vi "BlockAngle.vi"(8 "error in (no error)":errorcluster, 9 "Game ref":refnum<class "Game.lvclass">, 10 "Robot in":refnum<class "Robot.lvclass">, 11 "DefendGoalTactic in":refnum<class "DefendGoalTactic.lvclass">) -> (0 "error out":errorcluster, 2 "Robot out":refnum<class "Robot.lvclass">, 3 "DefendGoalTactic out":refnum<class "DefendGoalTactic.lvclass">)   [LabVIEW 2024, in "DefendGoalTactic.lvclass"]
uses:
  DefendGoalTactic.lvclass
  Game_class/Game.lvclass
  Robot_class/Robot.lvclass
  Game_class/Game.lvclass/Game.ctl
  Object_class/Object.lvclass/Object.ctl
  Team_class/Team.lvclass/Team.ctl
  Field_class/Field.lvclass/Field.ctl
  Robot_class/Robot.lvclass/Robot.ctl
  Game_class/Read BallRef.vi
  Game_class/Read FieldRef.vi
  Game_class/Read DefensiveTeam.vi
  Team_class/Read RobotRef.vi
  Field_class/Read ourGoalPosition.vi
  Object_class/Read position(x,y).vi
  Robot_class/Write dest_orientation.vi
  Robot_class/Write dest_x.vi
  Robot_class/Write dest_y.vi
  Robot_class/Write kick_x.vi
  Robot_class/Write kick_z.vi
  Ally_class/Ally.lvclass
  C:/Users/ROBOIME2/Documents/SSL ROBOIME/SSL_AI/Team_class/Team.lvclass
  Ball_class/Ball.lvclass
  C:/Users/ROBOIME2/Documents/SSL ROBOIME/SSL_AI/Object_class/Object.lvclass
  Field_class/Field.lvclass
  <vilib>/Analysis/NI_AALPro.lvlib
  Utilities_class/Utilities.lvclass
  <vilib>/Analysis/coordinate.llb/2D Cartesian Coordinate Rotation (Scalar).vi
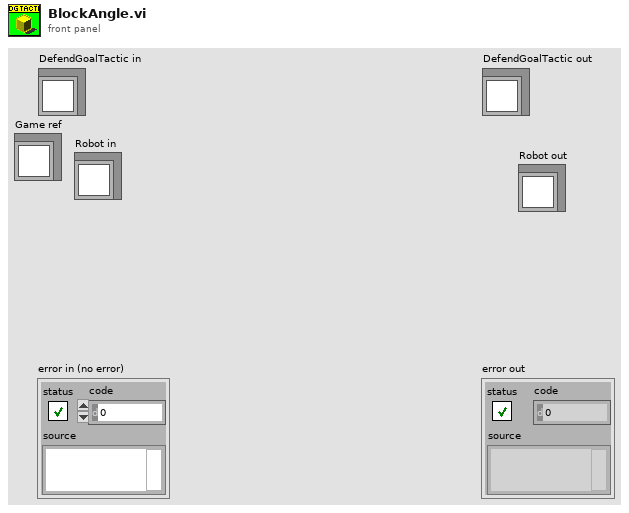
[diagram p1: front panel]
types:
  T1 = typedef "NewParameters.ctl" = cluster{"PenaltyDistance":dbl, "DistanceAttackerToBackBall":dbl, "Division":enum16{"Div B", "Div A"}, "DistanceToAvoidyEnemyRobot":dbl, "BallPlacementDistance":dbl, "DisatanceBehindBallToStealBall":dbl, "MaxDistanceToPositionKickoff":dbl, "BlockEnemyTarget":bool, "MaxStopVAng":dbl, "DistanceMarkerToEnemy":dbl, "IgnoreDribblerContact":bool, "DistanceToBeginEnemyPosession":dbl, "GoToBallWhenEnemyNotMoving":bool, "EnemyDistanceToReduceVelocity":dbl, "TurnOnEnemyDistanceToReduceVelocity":bool, "EnemyDistanceToShootOutBall":dbl, "DefenseKickBall":bool, "MoreKickToGoal? (0-0.3)":dbl, "ChipKickInEnemyField":bool, "ShootOutRobotId":dbl, "FieldLenghtDenominatorInShootOut":dbl, "AdjustPositionInBallPlacement":bool, "PowerGodPass":dbl, "VelocityAbortEnemyPos":dbl, "MaxDistToBeginPass":dbl, "MinDistToBeginPass":dbl, "VelocityInDirects":dbl, "BadDribblerIDs":i32[], "NewKickToDistanceAroundBall":dbl, "PowerAvoidColisionMarker":dbl, "DistanceToAvoidColisionMarker":dbl, "AvoidBallKick":dbl, "DistanceTryKick":dbl, "SuicideKickDIstance":dbl, "AdjustFirstKickDistance":dbl, "AvoidAimLessKick":dbl, "DistanceToAvoidyEnemyShootRobot ":dbl, "NumberOfMarkers":dbl, "PotField":bool, "PIDLateral":bool, "MinDistanceFirstKickX":dbl, "MinDistanceFirstKickY":dbl, "FractionOfDistToTouchGround\nAfterChipKick":dbl, "FractionOfKickxWhen\nComposedWithKickz":dbl, "Style":T2, "MoveInTurnState":bool, "DistFromEnemyToConsider\nMoveInTurnState":dbl, "CascadePID":bool, "TurnAroundParameters":cluster{"Radius":dbl, "Multiplier":dbl, "ChordAngle":dbl}, "SafeDriveVel":dbl, "DistanceToGoToBackBall":dbl, "minDistanceToNotFinish\nEnemyPossession":dbl, "OneTouchShot":cluster{"angleFactor":dbl, "maxAngle":dbl, "Attack":bool, "Defense":bool}, "OpenAngleToGoal":cluster{"minAngle":dbl, "maxAngle":dbl, "minEvaluation":dbl}, "ShotInterception":cluster{"shotSpeed":dbl, "minEnemySpeed":dbl, "maxEnemySpeed":dbl, "minEvaluation":dbl}, "AllyTeamArray":T3[], "maxDefendersNumber":i32, "Zone":cluster{"GuardPositionArray":dbl[][], "ZoneMidField":dbl[], "CenterForwardWidth":dbl}, "MinEvaluationToShoot":dbl, "PassInterception":cluster{"maxPassSpeed":dbl, "minPassSpeed":dbl, "minEnemySpeed":dbl, "chipPassDistance":dbl, "chipPassEvaluation":dbl, "minEvaluation":dbl, "maxEnemySpeed":dbl}, "PassDistance":cluster{"maxDistance":dbl, "minDistance":dbl}, "receiverSpeed":dbl, "maxBallSpeed":dbl, "slackTime":dbl, "Turning radius":dbl, "Turning v_ang":dbl, "AlignError":cluster{"Distance":dbl, "Orientation":dbl, "V_norm(m/s)":dbl, "V_ang (rad/s)":dbl}, "RobotRadius":dbl, "KickerDistance":dbl, "keeper angle  to cover goalpost":dbl, "a_slide":dbl, "a_roll":dbl, "k_switch":dbl}
  T2 = typedef "Style.ctl" = enum16{"Insanity", "Offensive", "Defensive"}
  T3 = typedef "AllyTeam.ctl" = enum16{"Keeper", "Defender", "Attacker"}
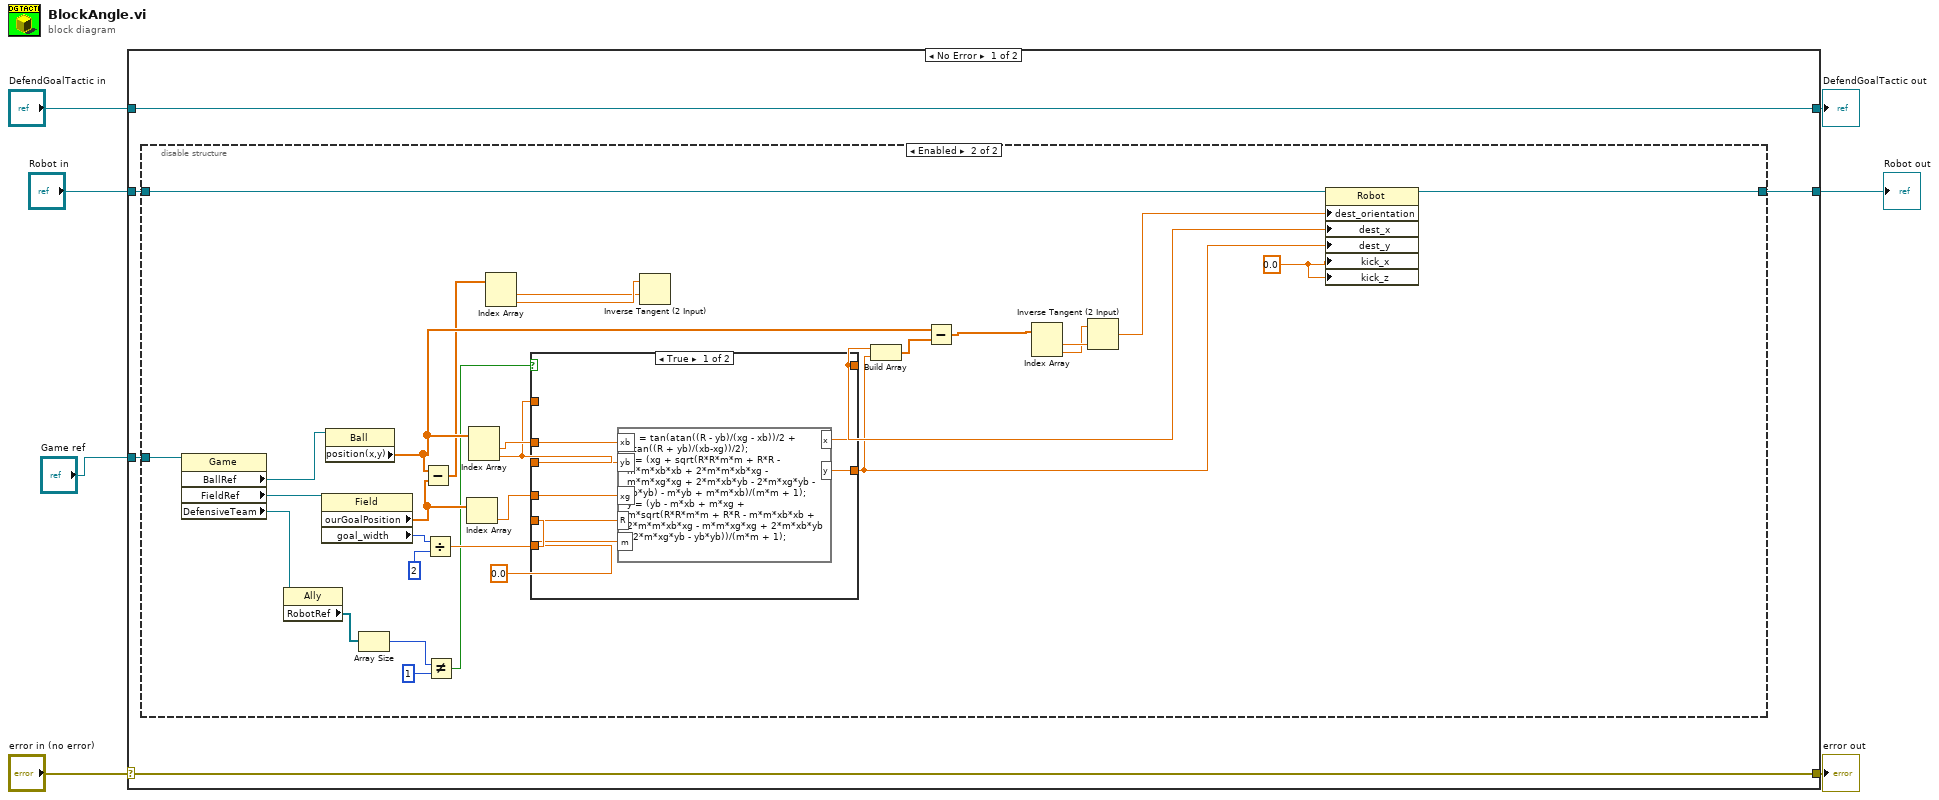
[diagram p0: block diagram]
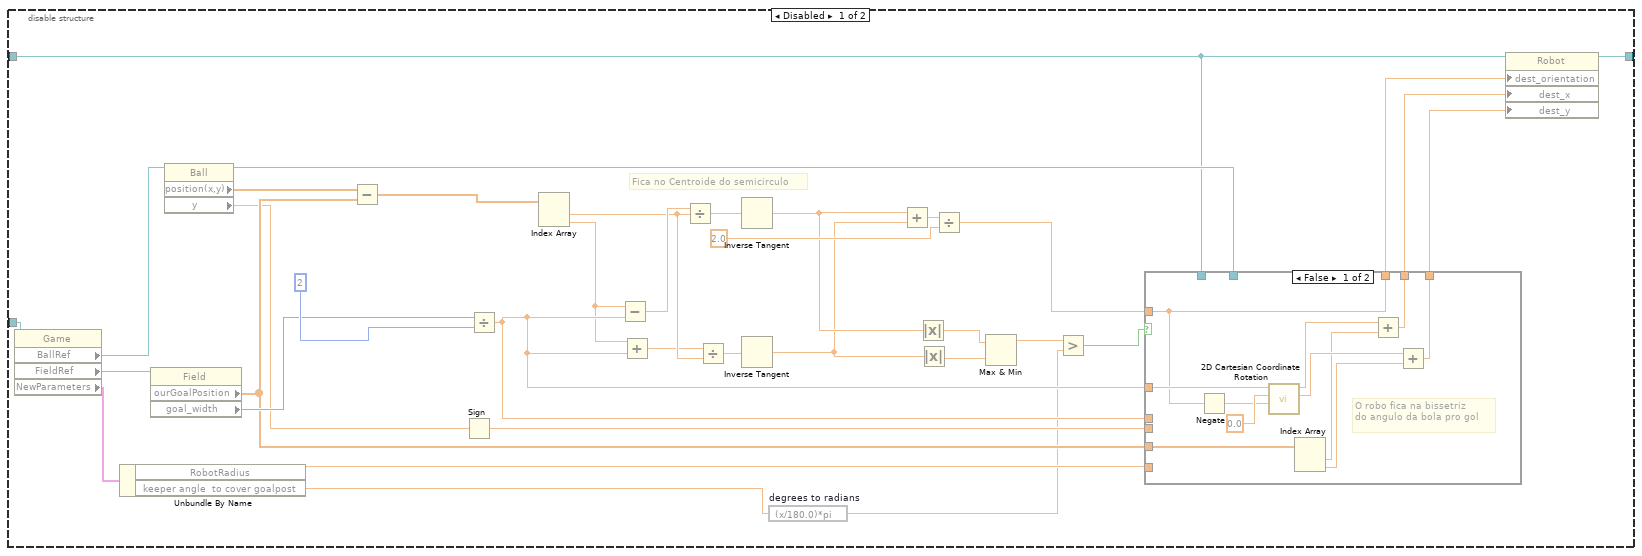
[diagram p2: hidden frame]
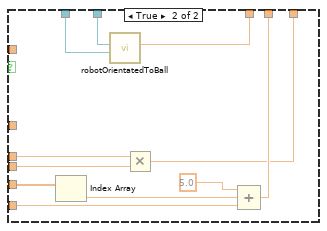
[diagram p3: hidden frame]
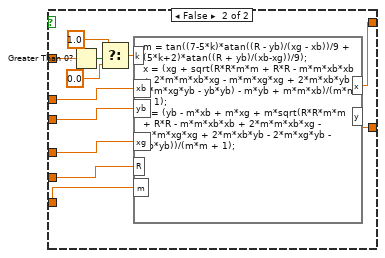
[diagram p4: hidden frame]
diagram:
  n1 = case shown="No Error" "error in (no error)" {
    selector: "error in (no error)" -> [w11 w122]
    tunnel: [w11 w122] -> w6
    tunnel: [w12 w121] -> w4
    tunnel: "DefendGoalTactic in" -> [w12 w121]
    tunnel: "Game ref" -> [w10 _]
    tunnel: "Robot in" -> [w8 w120]
    tunnel: [w9 w120] -> w1
    frame No Error {
      n2 = disable-structure shown="Enabled" {
        disable-tunnel: w10 -> [w23 w100]
        disable-tunnel: [w22 w88] -> w9
        disable-tunnel: w8 -> [w21 w89]
        frame Disabled {
          # "Fica no Centroide do semicirculo"
          n3 = property class="Game"(reference=w23) -> ("BallRef"=w48:refnum<class "Ball.lvclass">, "FieldRef"=w47:refnum<class "Field.lvclass">, "NewParameters"=w29:T1)  [unwired: 1 in, 2 out]
          n4 = Unbundle By Name(w29) -> ("RobotRadius"=w28:dbl, "keeper angle  to cover goalpost"=w13:dbl)
          n5 = property class="Field"(reference=w47) -> ("ourGoalPosition"=w35:dbl[], "goal_width"=w36:i32)  [unwired: 1 in, 2 out]
          n6 = property class="Ball"(reference=w48) -> (reference out=w30:refnum<class "Ball.lvclass">, "position(x,y)"=w46:dbl[], "y"=w25:dbl)  [unwired: 1 in, 1 out]
          n7 = Subtract(x=w46, y=w35) -> (x-y=w44:dbl[])
          n8 = Sign(1:w25) -> (0:w24:dbl)
          n9 = Divide(x=w36, y=2) -> (x/y=w27:dbl)
          n10 = Index Array(array=w44) -> (element #1=w42:dbl, element #2=w26:dbl)  [unwired: 2 in]
          n11 = Subtract(x=w26, y=w27) -> (x-y=w43:dbl)
          n12 = Add(x=w26, y=w27) -> (x+y=w41:dbl)
          n13 = Divide(x=w43, y=w42) -> (x/y=w45:dbl)
          n14 = Divide(x=w41, y=w42) -> (x/y=w40:dbl)
          n15 = Inverse Tangent(1:w45) -> (0:w20:dbl)
          n16 = Inverse Tangent(1:w40) -> (0:w19:dbl)
          n17 = expression code="(x/180.0)*pi" "degrees to radians"(w13) -> (w15:dbl)
          n18 = Add(x=w20, y=w19) -> (x+y=w38:dbl)
          n19 = Absolute Value(x=w20) -> (abs(x)=w18:dbl)
          n20 = Absolute Value(x=w19) -> (abs(x)=w17:dbl)
          n21 = Divide(x=w38, y=2.0) -> (x/y=w32:dbl)
          n22 = Max & Min(x=w18, y=w17) -> (max(x,y)=w16:dbl)  [unwired: 1 out]
          n23 = Greater?(x=w16, y=w15) -> (0:w14:bool)
          n24 = case shown="False" w14 {
            tunnel: w27 -> [w58 _]
            tunnel: w35 -> [w57 w67]
            tunnel: [w51 w64] -> w34
            tunnel: [w50 w61] -> w33
            tunnel: w32 -> [w49 _]
            tunnel: [w49 w69] -> w31
            tunnel: w30 -> [_ w70]
            tunnel: w28 -> [_ w68]
            tunnel: w27 -> [_ w62]
            tunnel: w24 -> [_ w63]
            tunnel: w21 -> [_ w60]
            frame False {
              # "O robo fica na bissetriz \ndo angulo da bola pro gol"
              n25 = Negate(x=w49) -> (-x=w54:dbl)
              n26 = call-poly <vilib>:"2D Cartesian Coordinate Rotation.vi"("theta"=w54, "y"=0.0, "x"=w58) -> ("y out"=w55:dbl, "x out"=w56:dbl)  [unwired: 6 in, 1 out]
              n27 = Index Array(array=w57) -> (element #1=w53:dbl, element #2=w52:dbl)  [unwired: 2 in]
              n28 = Add(x=w56, y=w53) -> (x+y=w51:dbl)
              n29 = Add(x=w55, y=w52) -> (x+y=w50:dbl)
            }
            frame True {
              n30 = Index Array(array=w67) -> (element=w66:dbl)  [unwired: 1 in]
              n31 = call "robotOrientatedToBall.vi"("Robot"=w60, "BallRef"=w70) -> ("Orientation"=w69:dbl)  [unwired: 7 in, 2 out]
              n32 = Multiply(x=w62, y=w63) -> (x*y=w61:dbl)
              n33 = Compound Arithmetic op=ADD(5.0 ("value"), w66, w68) -> (w64:dbl)
            }
          }
          n34 = property class="Robot"(reference=w21, "dest_orientation"=w31, "dest_x"=w34, "dest_y"=w33) -> (reference out=w22:refnum<class "Robot.lvclass">)  [unwired: 1 in, 1 out]
        }
        frame Enabled {
          w83 = 0.0 ("kick_x")
          n35 = property class="Game"(reference=w100) -> ("BallRef"=w98:refnum<class "Ball.lvclass">, "FieldRef"=w99:refnum<class "Field.lvclass">, "DefensiveTeam"=w76:refnum<class "Ally.lvclass">)  [unwired: 1 in, 2 out]
          n36 = property class="Ally"(reference=w76) -> ("RobotRef"=w75:refnum<class "Robot.lvclass">[])  [unwired: 1 in, 2 out]
          n37 = property class="Field"(reference=w99) -> ("ourGoalPosition"=w81:dbl[], "goal_width"=w95:i32)  [unwired: 1 in, 2 out]
          n38 = property class="Ball"(reference=w98) -> ("position(x,y)"=w82:dbl[])  [unwired: 1 in, 2 out]
          n39 = Array Size(array=w75) -> (size(s)=w74:i32)
          n40 = Subtract(x=w82, y=w81) -> (x-y=w80:dbl[])
          n41 = Divide(x=w95, y=2) -> (x/y=w93:dbl)
          n42 = Not Equal?(x=w74, y=1) -> (x != y?=w71:bool)
          n43 = Index Array(array=w81) -> (element=w96:dbl)  [unwired: 1 in]
          n44 = Index Array(array=w82) -> (element #1=w97:dbl, element #2=w72:dbl)  [unwired: 2 in]
          n45 = Index Array(array=w80) -> (element #1=w78:dbl, element #2=w79:dbl)  [unwired: 2 in]
          n46 = case shown="True" w71 {
            tunnel: w97 -> [w107 w119]
            tunnel: w72 -> [w106 w118]
            tunnel: w96 -> [w105 w117]
            tunnel: w93 -> [w104 w116]
            tunnel: [w103 w115] -> w86
            tunnel: [w102 w114] -> w85
            tunnel: 0.0 ("input variable") -> [w101 w113]
            tunnel: w72 -> [_ w108]
            frame True {
              n47 = formula code="m = tan(atan((R - yb)/(xg - xb))/2 + atan((R + yb)/(xb-xg))/2);\nx = (xg + sqrt(R*R*m*m + R*R - m*m*xb*xb + 2*m*m*xb*xg - m*m*xg*xg + 2*m*xb*yb - 2*m*xg*yb - yb*yb) - m*yb + m*m*xb)/(m*m + 1);\ny = (yb - m*xb + m*xg + m*sqrt(R*R*m*m + R*R - m*m*xb*xb + 2*m*m*xb*xg - m*m*xg*xg + 2*m*xb*yb - 2*m*xg*yb - yb*yb))/(m*m + 1);"("xb"=w107, "yb"=w106, "xg"=w105, "R"=w104, "m"=w101) -> ("x"=w103:dbl, "y"=w102:dbl)
            }
            frame False {
              n48 = Greater Than 0?(x=w108) -> (x > 0?=w112:bool)
              n49 = Select(t=1.0, s=w112, f=0.0 ("t")) -> (s? t:f=w109:dbl)
              n50 = formula code="m = tan((7-5*k)*atan((R - yb)/(xg - xb))/9 + (5*k+2)*atan((R + yb)/(xb-xg))/9);\nx = (xg + sqrt(R*R*m*m + R*R - m*m*xb*xb + 2*m*m*xb*xg - m*m*xg*xg + 2*m*xb*yb - 2*m*xg*yb - yb*yb) - m*yb + m*m*xb)/(m*m + 1);\ny = (yb - m*xb + m*xg + m*sqrt(R*R*m*m + R*R - m*m*xb*xb + 2*m*m*xb*xg - m*m*xg*xg + 2*m*xb*yb - 2*m*xg*yb - yb*yb))/(m*m + 1);"("xb"=w119, "yb"=w118, "xg"=w117, "R"=w116, "m"=w113, "k"=w109) -> ("x"=w115:dbl, "y"=w114:dbl)
            }
          }
          n51 = Inverse Tangent (2 Input)(1:w78, 2:w79) -> ()  [unwired: 1 out]
          n52 = Build Array(w86, w85) -> (w92:dbl[])
          n53 = Subtract(x=w82, y=w92) -> (x-y=w77:dbl[])
          n54 = Index Array(array=w77) -> (element #1=w91:dbl, element #2=w90:dbl)  [unwired: 2 in]
          n55 = Inverse Tangent (2 Input)(1:w91, 2:w90) -> (0:w87:dbl)
          n56 = property class="Robot"(reference=w89, "dest_orientation"=w87, "dest_x"=w86, "dest_y"=w85, "kick_x"=w83, "kick_z"=w83) -> (reference out=w88:refnum<class "Robot.lvclass">)  [unwired: 1 in, 1 out]
        }
      }
    }
    frame Error {
    }
  }
  "error out" <- w6
  "DefendGoalTactic out" <- w4
  "Robot out" <- w1
